vi "Teleop.vi"(10 "Match Info":T1={"Autonomous Elapsed Seconds"=0.0, "TeleOp Elapsed Seconds"=0.0, "Disabled Elapsed Seconds"=0.0, "Visited Autonomous"=FALSE, "Visited TeleOp"=FALSE, "Visited Disabled"=FALSE, "Autonomous Settings"={"Autonomous Style"=enum."Independent", "VI Refnum"=refnum}}, 11 "Call Context":T2) -> ()   [LabVIEW 2019]
doc: "This VI is called for each enabled TeleOp packet received from the DS. It is typically used to read from joysticks and other inputs and update I/O or setpoints for timed control loops. It should complete and return within 20 milliseconds or risk missing DS packets."
uses:
  <vilib>/Rock Robotics/WPI/DriverStation/WPI_DriverStationDerivedRobotMode.ctl
  <vilib>/Rock Robotics/WPI/DriverStation/WPI_DriverStationMatch Info.ctl
  Framework/Robot Global Data.vi
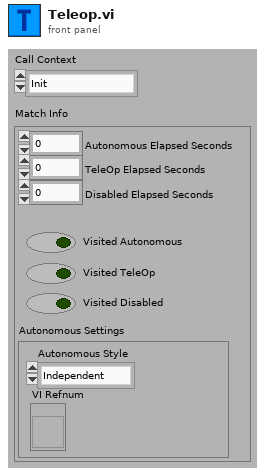
[diagram p1: front panel]
types:
  T1 = typedef "WPI_DriverStationMatch Info.ctl" = cluster{"Autonomous Elapsed Seconds":dbl, "TeleOp Elapsed Seconds":dbl, "Disabled Elapsed Seconds":dbl, "Visited Autonomous":bool, "Visited TeleOp":bool, "Visited Disabled":bool, "Autonomous Settings":cluster{"Autonomous Style":enum16{"Iterative", "Independent"}, "VI Refnum":refnum<vi>}}
  T2 = typedef "WPI_DriverStationDerivedRobotMode.ctl" = enum16{"Init", "Execute", "Stop"}
  T3 = typedef "Command Status Info.ctl" = cluster{"Name":string, "Status":T4, "notifier out":T5}
  T4 = typedef "Completion Status.ctl" = enum16{"Successful", "Aborted", "Incomplete"}
  T5 = typedef "Completion Notifier.ctl" = refnum<notifier>
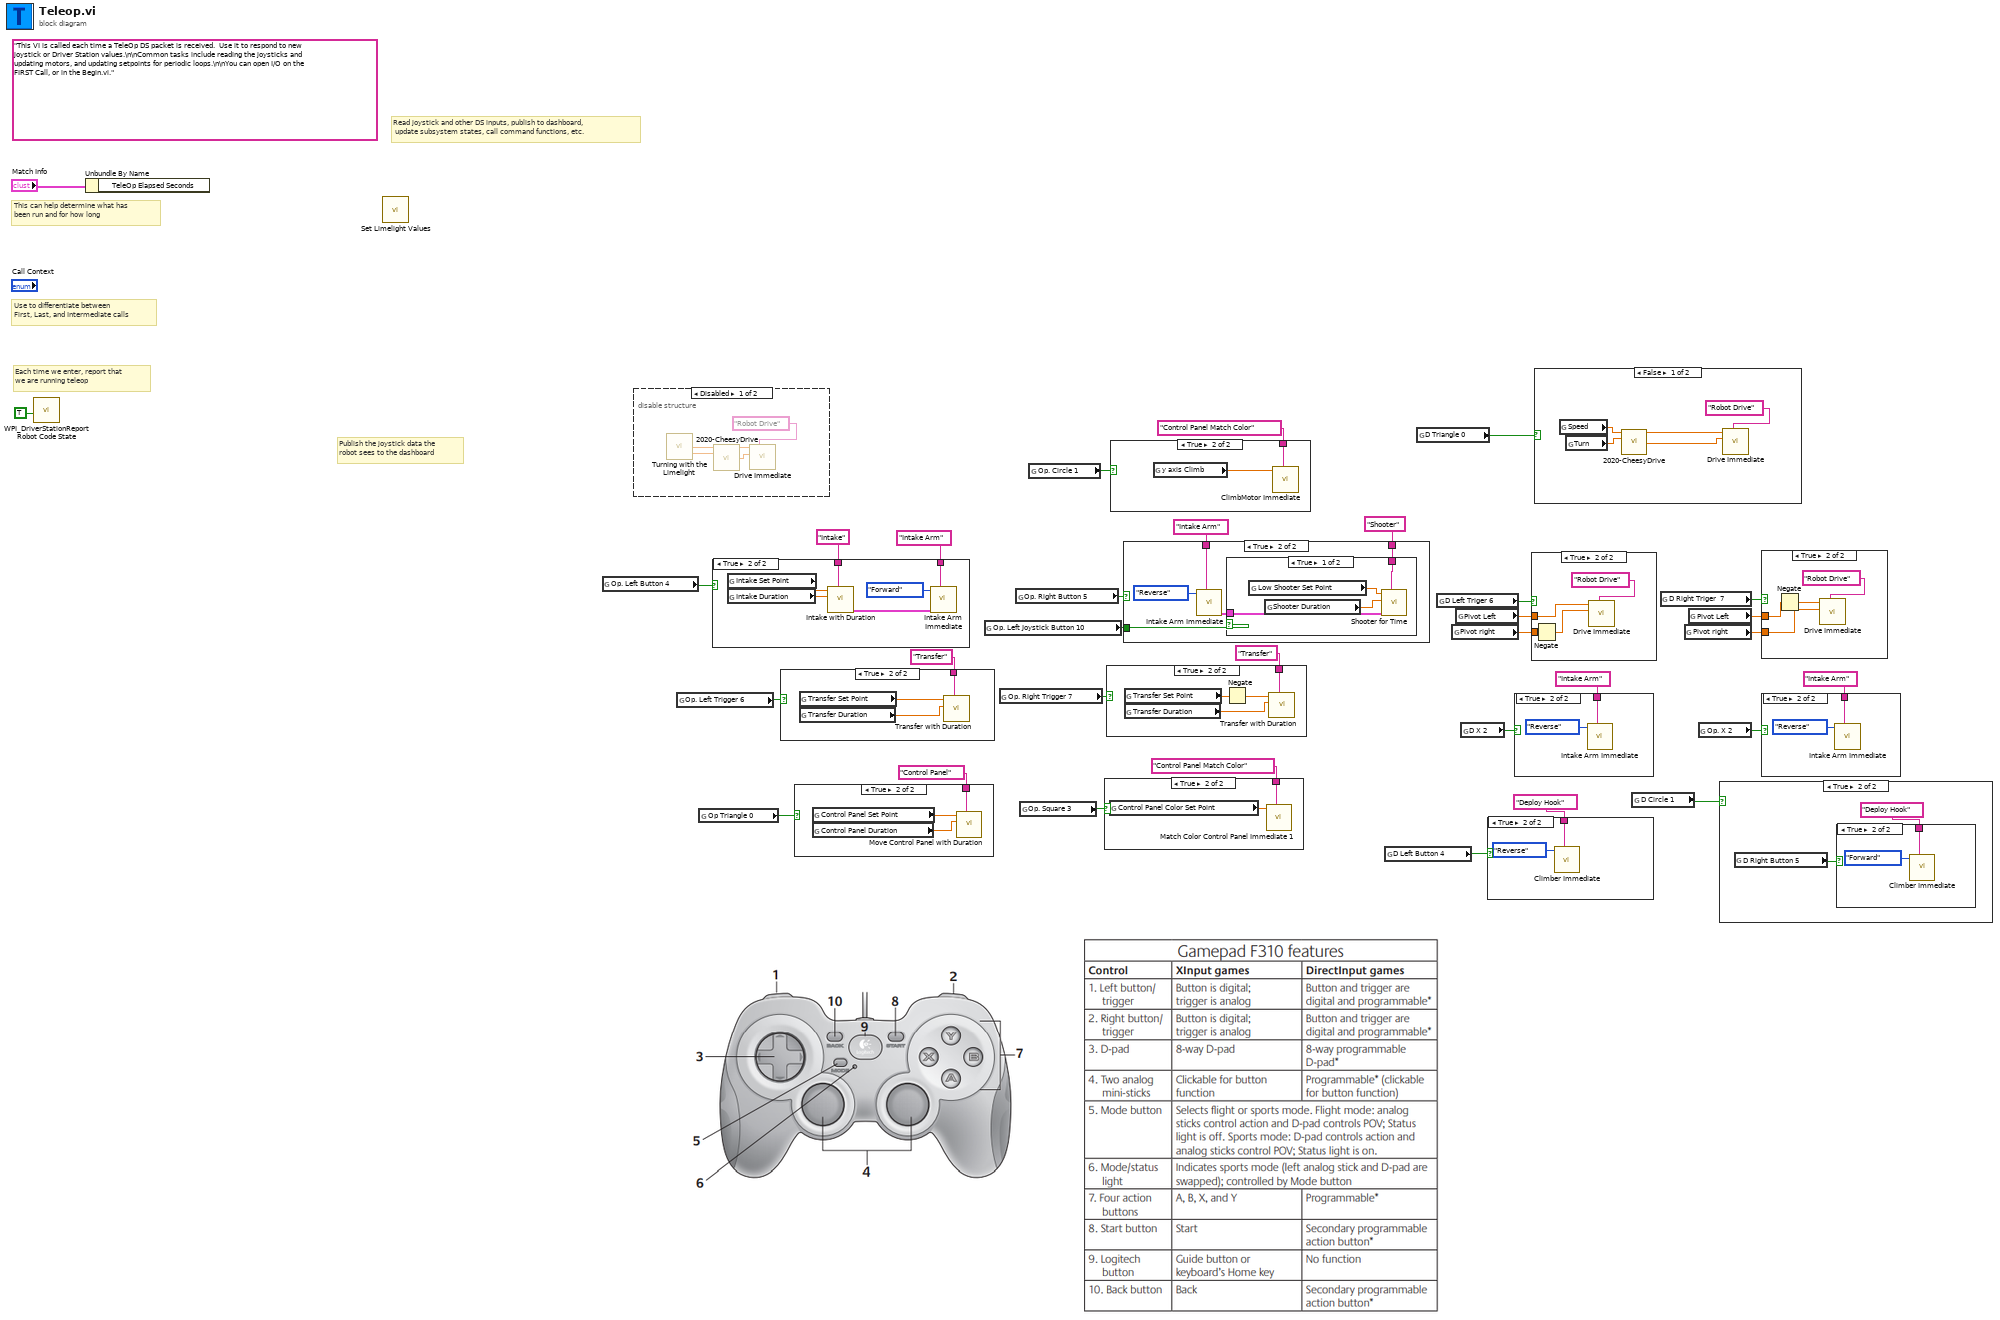
[diagram p0: block diagram]
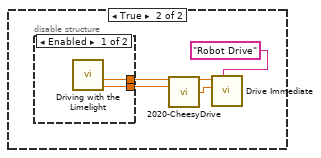
[diagram p8: hidden frame]
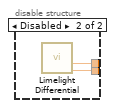
[diagram p9: hidden frame]
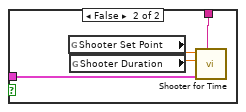
[diagram p18: hidden frame]
diagram:
  (unwired) "This VI is called each time a TeleOp DS packet is received.  Use it to respond to new joystick or Driver Station values.\n\nCommon tasks include reading the joysticks and updating motors, and updating setpoints for periodic loops.\n\nYou can open I/O on the FIRST Call, or in the Begin.vi."
  # "Publish the joystick data the\nrobot sees to the dashboard"
  # "Read joystick and other DS inputs, publish to dashboard,\n update subsystem states, call command functions, etc."
  # "Each time we enter, report that\nwe are running teleop"
  # "Use to differentiate between\nFirst, Last, and Intermediate calls"
  # "This can help determine what has\nbeen run and for how long"
  n1 = call <vilib>:"WPI_DriverStationReport Robot Code State.vi"("TeleOp"=TRUE ("Autonomous")) -> ()  [unwired: 10 in, 1 out]
  n2 = Unbundle By Name("Match Info") -> ()  [unwired: 1 out]
  n3 = call "Set Limelight Values.vi"() -> ()  [unwired: 12 in]
  n4 = global read "Robot Global Data.vi" "Op. Left Button 4"() -> (w31:bool)
  n5 = disable-structure shown="Disabled" {
    frame Disabled {
      n6 = call "Turning with the Limelight.vi"() -> ("TurnCommand"=w37:dbl, "Speed Command"=w38:dbl)  [unwired: 9 in, 1 out]
      n7 = call "2020-CheesyDrive.vi"("Throttle"=w38, "Wheel"=w37) -> ("Left PWM"=w36:dbl, "Right PWM"=w35:dbl)  [unwired: 12 in]
      n8 = call "Drive Immediate.vi"("Description"="Robot Drive", "Right Setpoint"=w35, "Left Setpoint"=w36) -> ()  [unwired: 8 in, 1 out]
    }
    frame Enabled {
    }
  }
  n9 = global read "Robot Global Data.vi" "Op. Left Trigger 6"() -> (w25:bool)
  n10 = global read "Robot Global Data.vi" "Op Triangle 0"() -> (w18:bool)
  n11 = case shown="True" w31 {
    tunnel: "Intake" ("refnum name") -> [_ w44]
    tunnel: "Intake Arm" ("refnum name") -> [_ w40]
    frame False {
    }
    frame True {
      n12 = global read "Robot Global Data.vi" "Intake Set Point"() -> (w43:dbl)
      n13 = global read "Robot Global Data.vi" "Intake Duration"() -> (w42:dbl)
      n14 = call "Intake with Duration.vi"("Description"=w44, "Duration (s)"=w42, "Setpoint"=w43) -> ("Command Info Out"=w39:T3)  [unwired: 8 in]
      n15 = call "Intake Arm Immediate.vi"("Description"=w40, "Command Info In"=w39, "Relay Value"=enum16{"Off", "On", "Forward", "Reverse"}."Forward") -> ()  [unwired: 8 in, 1 out]
    }
  }
  n16 = case shown="True" w25 {
    tunnel: "Transfer" ("refnum name") -> [_ w47]
    frame False {
    }
    frame True {
      n17 = global read "Robot Global Data.vi" "Transfer Set Point"() -> (w46:dbl)
      n18 = global read "Robot Global Data.vi" "Transfer Duration"() -> (w45:dbl)
      n19 = call "Transfer with Duration.vi"("Description"=w47, "Duration (s)"=w45, "Setpoint"=w46) -> ()  [unwired: 8 in, 1 out]
    }
  }
  n20 = case shown="True" w18 {
    tunnel: "Control Panel" ("refnum name") -> [_ w50]
    frame False {
    }
    frame True {
      n21 = global read "Robot Global Data.vi" "Control Panel Set Point"() -> (w49:dbl)
      n22 = global read "Robot Global Data.vi" "Control Panel Duration"() -> (w48:dbl)
      n23 = call "Move Control Panel with Duration.vi"("Description"=w50, "Duration (s)"=w48, "Setpoint"=w49) -> ()  [unwired: 8 in, 1 out]
    }
  }
  n24 = global read "Robot Global Data.vi" "Op. Left Joystick Button 10"() -> (w1:bool)
  n25 = global read "Robot Global Data.vi" "Op. Right Trigger 7"() -> (w26:bool)
  n26 = global read "Robot Global Data.vi" "Op. Right Button 5"() -> (w27:bool)
  n27 = global read "Robot Global Data.vi" "Op. Square 3"() -> (w15:bool)
  n28 = global read "Robot Global Data.vi" "Op. Circle 1"() -> (w3:bool)
  n29 = case shown="True" w15 {
    tunnel: "Control Panel Match Color" ("refnum name") -> [_ w52]
    frame False {
    }
    frame True {
      n30 = global read "Robot Global Data.vi" "Control Panel Color Set Point"() -> (w51:dbl)
      n31 = call "Match Color Control Panel Immediate 1.vi"("Description"=w52, "Setpoint"=w51) -> ()  [unwired: 9 in, 1 out]
    }
  }
  n32 = case shown="True" w26 {
    tunnel: "Transfer" ("refnum name") -> [_ w56]
    frame False {
    }
    frame True {
      n33 = global read "Robot Global Data.vi" "Transfer Set Point"() -> (w54:dbl)
      n34 = global read "Robot Global Data.vi" "Transfer Duration"() -> (w53:dbl)
      n35 = Negate(x=w54) -> (-x=w55:dbl)
      n36 = call "Transfer with Duration.vi"("Description"=w56, "Duration (s)"=w53, "Setpoint"=w55) -> ()  [unwired: 8 in, 1 out]
    }
  }
  n37 = case shown="True" w3 {
    tunnel: "Control Panel Match Color" ("refnum name") -> [_ w58]
    frame False {
    }
    frame True {
      n38 = global read "Robot Global Data.vi" "y axis Climb"() -> (w57:dbl)
      n39 = call "ClimbMotor Immediate.vi"("Description"=w58, "Setpoint"=w57) -> ()  [unwired: 9 in, 1 out]
    }
  }
  n40 = case shown="True" w27 {
    tunnel: "Shooter" ("refnum name") -> [_ w63]
    tunnel: "Intake Arm" ("refnum name") -> [_ w60]
    tunnel: w1 -> [_ w59]
    frame False {
    }
    frame True {
      n41 = call "Intake Arm Immediate.vi"("Description"=w60, "Relay Value"=enum16{"Off", "On", "Forward", "Reverse"}."Reverse") -> ("Command Info Out"=w61:T3)  [unwired: 9 in]
      n42 = case shown="True" w59 {
        tunnel: w63 -> [w67 w71]
        tunnel: w61 -> [w65 w68]
        frame True {
          n43 = global read "Robot Global Data.vi" "Low Shooter Set Point"() -> (w64:dbl)
          n44 = global read "Robot Global Data.vi" "Shooter Duration"() -> (w66:dbl)
          n45 = call "Shooter for Time.vi"("Description"=w67, "Command Info In"=w65, "Duration (s)"=w66, "Setpoint"=w64) -> ()  [unwired: 7 in, 1 out]
        }
        frame False {
          n46 = global read "Robot Global Data.vi" "Shooter Set Point"() -> (w70:dbl)
          n47 = global read "Robot Global Data.vi" "Shooter Duration"() -> (w69:dbl)
          n48 = call "Shooter for Time.vi"("Description"=w71, "Command Info In"=w68, "Duration (s)"=w69, "Setpoint"=w70) -> ()  [unwired: 7 in, 1 out]
        }
      }
    }
  }
  n49 = global read "Robot Global Data.vi" "D Left Button 4"() -> (w8:bool)
  n50 = global read "Robot Global Data.vi" "D Triangle 0"() -> (w9:bool)
  n51 = global read "Robot Global Data.vi" "D Left Triger 6"() -> (w23:bool)
  n52 = global read "Robot Global Data.vi" "Pivot right"() -> (w12:dbl)
  n53 = global read "Robot Global Data.vi" "Pivot Left"() -> (w13:dbl)
  n54 = global read "Robot Global Data.vi" "D X 2"() -> (w16:bool)
  n55 = case shown="True" w8 {
    tunnel: "Deploy Hook" ("refnum name") -> [_ w72]
    frame False {
    }
    frame True {
      n56 = call "Climber Immediate.vi"("Description"=w72, "Value"=enum16{"Off", "On", "Forward", "Reverse"}."Reverse" ("Relay Value")) -> ()  [unwired: 9 in, 1 out]
    }
  }
  n57 = case shown="True" w16 {
    tunnel: "Intake Arm" ("refnum name") -> [_ w74]
    frame False {
    }
    frame True {
      n58 = call "Intake Arm Immediate.vi"("Description"=w74, "Relay Value"=enum16{"Off", "On", "Forward", "Reverse"}."Reverse") -> ()  [unwired: 9 in, 1 out]
    }
  }
  n59 = case shown="True" w23 {
    tunnel: w13 -> [_ w78]
    tunnel: w12 -> [_ w77]
    frame False {
    }
    frame True {
      n60 = Negate(x=w77) -> (-x=w76:dbl)
      n61 = call "Drive Immediate.vi"("Description"="Robot Drive", "Right Setpoint"=w76, "Left Setpoint"=w78) -> ()  [unwired: 8 in, 1 out]
    }
  }
  n62 = case shown="False" w9 {
    frame False {
      n63 = global read "Robot Global Data.vi" "Speed"() -> (w81:dbl)
      n64 = global read "Robot Global Data.vi" "Turn"() -> (w82:dbl)
      n65 = call "2020-CheesyDrive.vi"("Throttle"=w81, "Wheel"=w82) -> ("Left PWM"=w83:dbl, "Right PWM"=w84:dbl)  [unwired: 12 in]
      n66 = call "Drive Immediate.vi"("Description"="Robot Drive", "Right Setpoint"=w84, "Left Setpoint"=w83) -> ()  [unwired: 8 in, 1 out]
    }
    frame True {
      n67 = disable-structure shown="Enabled" {
        disable-tunnel: [w91 w92] -> w85
        disable-tunnel: [w90 w93] -> w86
        frame Enabled {
          n68 = call "Driving with the Limelight.vi"() -> ("TurnCommand"=w91:dbl, "SpeedCommand"=w90:dbl)  [unwired: 9 in, 1 out]
        }
        frame Disabled {
          n69 = call "Limelight Differential.vi"() -> ("DriveCommand"=w92:dbl, "SteerCommand"=w93:dbl)  [unwired: 9 in, 1 out]
        }
      }
      n70 = call "2020-CheesyDrive.vi"("Throttle"=w86, "Wheel"=w85) -> ("Left PWM"=w88:dbl, "Right PWM"=w89:dbl)  [unwired: 12 in]
      n71 = call "Drive Immediate.vi"("Description"="Robot Drive", "Right Setpoint"=w89, "Left Setpoint"=w88) -> ()  [unwired: 8 in, 1 out]
    }
  }
  n72 = global read "Robot Global Data.vi" "D Circle 1"() -> (w2:bool)
  n73 = global read "Robot Global Data.vi" "D Right Triger  7"() -> (w22:bool)
  n74 = global read "Robot Global Data.vi" "Pivot right"() -> (w10:dbl)
  n75 = global read "Robot Global Data.vi" "Pivot Left"() -> (w11:dbl)
  n76 = global read "Robot Global Data.vi" "Op. X 2"() -> (w6:bool)
  n77 = case shown="True" w2 {
    frame False {
    }
    frame True {
      n78 = global read "Robot Global Data.vi" "D Right Button 5"() -> (w94:bool)
      n79 = case shown="True" w94 {
        tunnel: "Deploy Hook" ("refnum name") -> [_ w96]
        frame False {
        }
        frame True {
          n80 = call "Climber Immediate.vi"("Description"=w96, "Value"=enum16{"Off", "On", "Forward", "Reverse"}."Forward" ("Relay Value")) -> ()  [unwired: 9 in, 1 out]
        }
      }
    }
  }
  n81 = case shown="True" w22 {
    tunnel: w11 -> [_ w100]
    tunnel: w10 -> [_ w99]
    frame False {
    }
    frame True {
      n82 = Negate(x=w100) -> (-x=w98:dbl)
      n83 = call "Drive Immediate.vi"("Description"="Robot Drive", "Right Setpoint"=w99, "Left Setpoint"=w98) -> ()  [unwired: 8 in, 1 out]
    }
  }
  n84 = case shown="True" w6 {
    tunnel: "Intake Arm" ("refnum name") -> [_ w102]
    frame False {
    }
    frame True {
      n85 = call "Intake Arm Immediate.vi"("Description"=w102, "Relay Value"=enum16{"Off", "On", "Forward", "Reverse"}."Reverse") -> ()  [unwired: 9 in, 1 out]
    }
  }
